vi "Antrenare neuroni ghicire simboluri.vi"(1 "Pixel patterns":bool[][](array[boolean])) -> (0 "Response":bool[](array[boolean]))   [LabVIEW 2025]
uses:
  <vilib>/National Instruments/NI Super Simple Neural Networks/Types/Teaching Settings.ctl
  <vilib>/National Instruments/NI Super Simple Neural Networks/Types/Error Evaluation.ctl
  <vilib>/National Instruments/NI Super Simple Neural Networks/API/Create 1 Hidden Layer.vi
  <vilib>/National Instruments/NI Super Simple Neural Networks/Neural Network.lvclass
panel:
  out "Solution Found":bool
  out "Waveform Chart":dbl[](graph)
  # "!"
  # "@"
  # "#"
  # "$"
  # "%"
  # "^"
  # "&"
  # "*"
  # "("
  # ")"
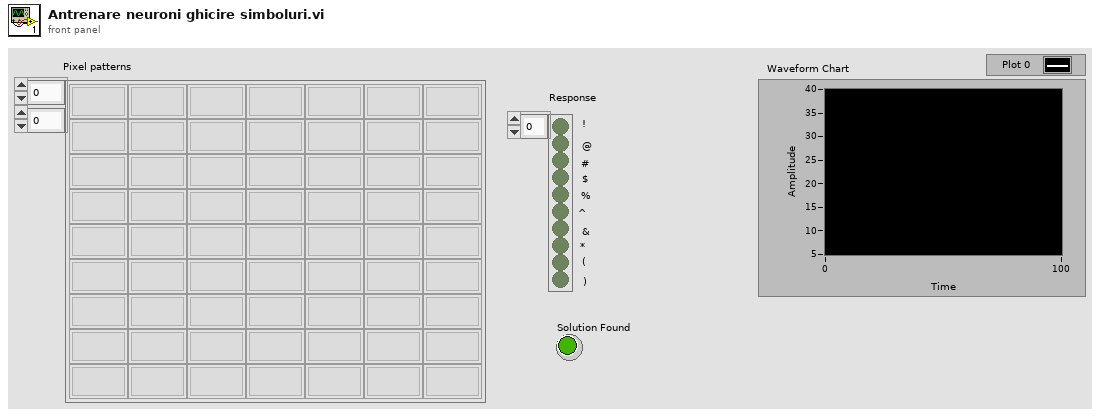
[diagram p1: front panel]
types:
  T1 = typedef "Neural Network.lvclass/Teaching Settings.ctl" = cluster{"Max Epocs":u64, "Error Goal":dbl, "Max Time (s)":dbl, "Error Evaluation":T2, "# Vectors per Iteration":i32}
  T2 = typedef "Neural Network.lvclass/Error Evaluation.ctl" = enum16{"Over Both Sets", "Over Validation Set", "Over Teaching Set"}
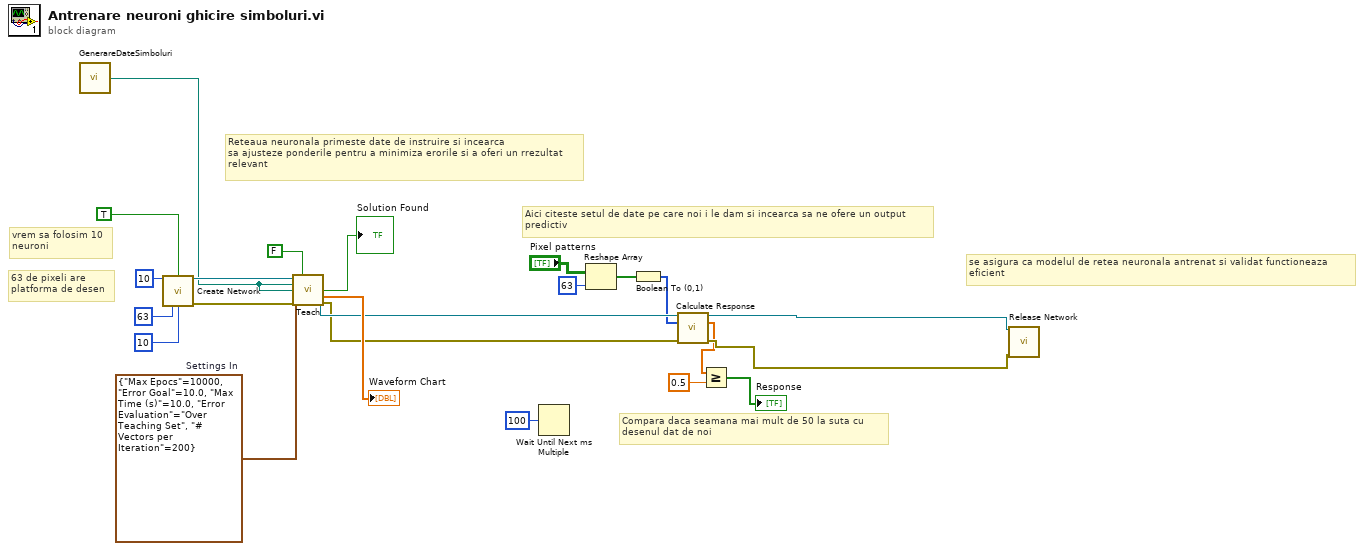
[diagram p0: block diagram]
diagram:
  w17 = T1 {"Max Epocs"=10000, "Error Goal"=10.0, "Max Time (s)"=10.0, "Error Evaluation"=enum."Over Teaching Set", "# Vectors per Iteration"=200}  # Settings In
  # "Compara daca seamana mai mult de 50 la suta cu \ndesenul dat de noi"
  # "Aici citeste setul de date pe care noi i le dam si incearca sa ne ofere un output\npredictiv"
  # "se asigura ca modelul de retea neuronala antrenat si validat functioneaza \neficient"
  # "Reteaua neuronala primeste date de instruire si incearca\nsa ajusteze ponderile pentru a minimiza erorile si a oferi un rrezultat\nrelevant"
  # "63 de pixeli are \nplatforma de desen"
  # "vrem sa folosim 10\nneuroni"
  n1 = call "GenerareDateSimboluri.vi"() -> ("path"=w9:path)
  n2 = call-poly <vilib>:"Create Network.vi"("1st Hidden Layer Neurons"=u32 10, "Add Bias Inputs (True)"=TRUE, "# Inputs"=u32 63, "Output Neurons/Outputs"=u32 10) -> ("Neural Network Out"=w19:refnum<class "Neural Network.lvclass">, "Error Out"=w18:errorcluster)  [unwired: 10 in]
  n3 = call <vilib>:"Teach.vi"("Neural Network In"=w19, "Enable Growing/Prunning"=FALSE, "Teaching Set Path In"=w9, "Validation Set Path In"=w9, "Settings In"=w17, "Error In"=w18) -> ("Neural Network Out"=w15:refnum<class "Neural Network.lvclass">, "Solution Found"=→"Solution Found":bool, "Error Trend Out"=→"Waveform Chart":dbl[], "Error Out"=w14:errorcluster)  [unwired: 5 in, 1 out]
  n4 = Wait Until Next ms Multiple(millisecond multiple=u32 100) -> ()  [unwired: 1 out]
  n5 = Reshape Array("Pixel patterns", 63 ("dimension size")) -> (w5:bool[])
  n6 = Boolean To (0,1)(Boolean=w5) -> (0, 1=w4:i16[])
  n7 = call <vilib>:"Calculate Response.vi"("Neural Network In"=w15, "Inputs"=w4, "Error In"=w14) -> ("Neural Network Out"=w13:refnum<class "Neural Network.lvclass">, "Outputs"=w2:dbl[], "Error Out"=w12:errorcluster)  [unwired: 10 in]
  n8 = Greater Or Equal?(x=w2, y=0.5) -> (x >= y?=→"Response":bool[])
  n9 = call <vilib>:"Release Network.vi"("Neural Network"=w13, "Error In"=w12) -> ()  [unwired: 13 in, 1 out]
